vi "Build Application.vi"(8 "error in (no error)":errorcluster, 11 "PostBuildSupport in":refnum<class "PostBuildSupport.lvclass">) -> (0 "error out":errorcluster, 3 "PostBuildSupport out":refnum<class "PostBuildSupport.lvclass">)   [LabVIEW 2019, in "PostBuildSupport.lvclass"]
uses:
  PostBuildSupport.lvclass
  PostBuildSupport.lvclass/PostBuildSupport.ctl
  <vilib>/AppBuilder/AB_API_Simple/Build (path).vi
  <vilib>/AppBuilder/AB_API_Simple/NI_App_Builder_API.lvlib
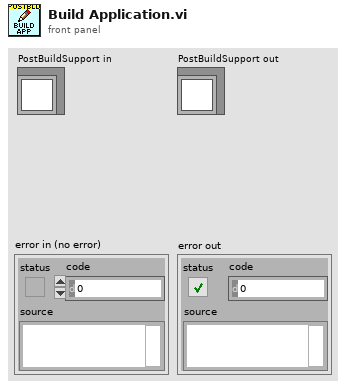
[diagram p1: front panel]
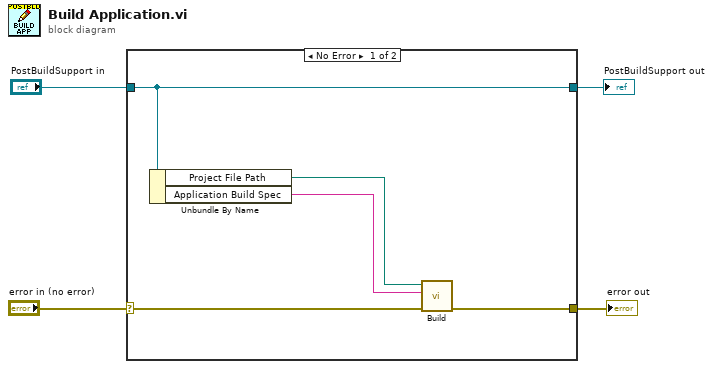
[diagram p0: block diagram]
diagram:
  n1 = case shown="No Error" "error in (no error)" {
    selector: "error in (no error)" -> [w8 w11]
    tunnel: "PostBuildSupport in" -> [w7 w10]
    tunnel: [w9 w11] -> w2
    tunnel: [w7 w10] -> w1
    frame No Error {
      n2 = Unbundle By Name(w7) -> ("Project File Path"=w5:path, "Application Build Spec"=w6:string)
      n3 = call-poly <vilib>:"Build.vi"("error in (no error)"=w8, "Name of build specification (if empty: build all)"=w6, "Path to project"=w5) -> ("error out"=w9:errorcluster)  [unwired: 7 in, 1 out]
    }
    frame Error {
    }
  }
  "error out" <- w2
  "PostBuildSupport out" <- w1
